vi "Multi Publisher.vi"() -> ()   [LabVIEW 2021]
uses:
  New Connection Request.ctl
  CIFChannels/CIFChannels.lvclass
  CIF_NIChn/FIFO_DAQ/CIF_NIChn_Fifo_DAQ.lvclass
  D:/dev/Packages/Channel_Manager/src/CIFChannels/CIFChannels.lvclass
  D:/dev/Packages/Channel_Manager/src/CIF_NIChn/NIChn/CIF_NIChn.lvclass
  CIFChannels/Typedef/Direction.ctl
  ChannelCommon/typedef/FIFO Config.ctl
  CIFChannels/CIFChannels.lvclass/CIFChannels.ctl
  ChannelCommon/typedef/Datatype Waveform.ctl
  ChannelCommon/typedef/TimeStamps.ctl
  CIF_NIChn/FIFO_DAQ/CIF_NIChn_Fifo_DAQ.lvclass/CIF_NIChn_Fifo_DAQ.ctl
  CIF_NIChn/NIChn/CIF_NIChn.lvclass/CIF_NIChn.ctl
  CIFChannels/Accessors/Write FIFO Retry on Timeout.vi
  CIFChannels/Accessors/Read Name.vi
  <vilib>/CIF Foundation/CIF Utilities/DataTypes/Flatten U64.vi
  CIF_NIChn/FIFO_DAQ/SubVIs/Core Write DAQ FIFO.vi
  ChannelCommon/Utilities/Reset Waveform DVRs.vi
  CIF_NIChn/FIFO_DAQ/SubVIs/Core Write DAQ DVR FIFO.vi
  ChannelCommon/Utilities/Get Waveform DVRs.vi
  CIFChannels/Accessors/Read FIFO Retry on Timeout.vi
  <vilib>/CIF Foundation/CIF Channels/CIFChannels/Top Level/Write U8 Array.vi
  CIF_NIChn/NIChn/Accessors/Read CIF Channel.vi
  CIF_NIChn/NIChn/Accessors/Write CIF Channel.vi
  CIF_NIChn/FIFO_DAQ/SubVIs/Flatten.vi
  CIFChannels/Accessors/Read FIFO Header.vi
  <vilib>/CIF Foundation/CIF Channels/CIFChannels/SubVIs/Get dll Path.vi
  <vilib>/CIF Foundation/CIF Channels/CIFChannels/SubVIs/Get Requested Size.vi
  ChannelCommon/CIFFIFO/Flatten/DVR Flatten.vi
  CIFChannels/Utilities/Create Flattened FIFO Header.vi
  ChannelCommon/Utilities/Flatten Header.vi
  CIFChannels/Utilities/Update FIFO Header.vi
  <vilib>/CIF Foundation/CIF Utilities/DataTypes/Flatten I64.vi
  <vilib>/CIF Foundation/CIF Utilities/Time/System Time/Get System Time.vi
  <vilib>/CIF Foundation/CIF Utilities/Time/System Time/LabVIEW Time to TAI Time.vi
  ChannelCommon/ChannelCommon.lvlib
panel:
  in  "Remove Pub":string
  in  "Remove":bool
  in  "stop":bool
  in  "Add":bool
  in  "New Sub":T1
  out "New Pub":string
  out "error out":errorcluster
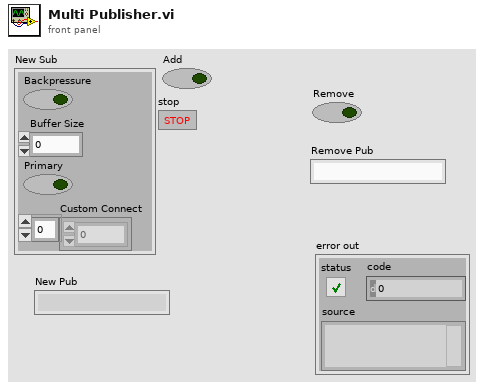
[diagram p1: front panel]
types:
  T1 = typedef "New Connection Request.ctl" = cluster{"Backpressure":bool, "Buffer Size":u64, "Primary":bool, "Custom Connect":u8[]}
  T2 = typedef "ChannelCommon.lvlib/TimeStamps.ctl" = cluster{"ClockID":u8, "T0":i64, "T_Out":i64}
  T3 = typedef "ChannelCommon.lvlib/Datatype Waveform.ctl" = cluster{"measurement":dbl[], "dT":dbl, "Timestamp":i64, "Read Lock":bool}
  T4 = typedef "ChannelCommon.lvlib/FIFO Config.ctl" = cluster{"Max Bytes/Msg":u64, "Max Msg/FIFO":u64, "Flags":u64}
  T5 = typedef "CIFChannels.lvclass/Direction.ctl" = enum16{"Publisher", "Subscriber"}
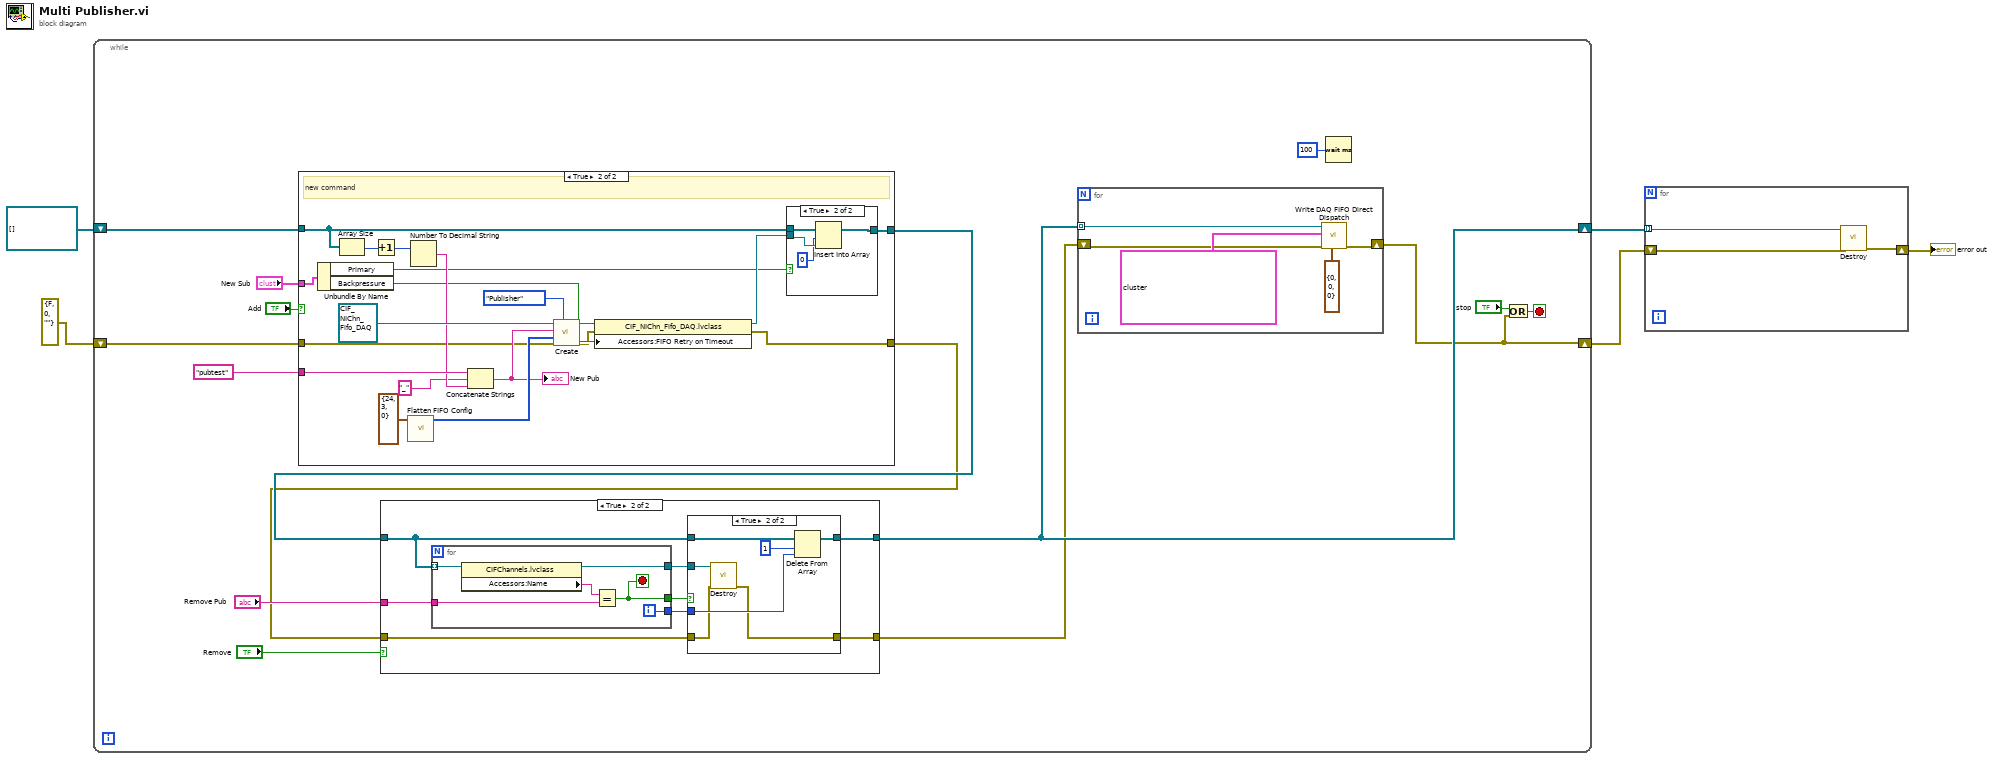
[diagram p0: block diagram]
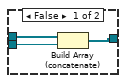
[diagram p5: hidden frame]
diagram:
  n1 = while {
    shift-right: [w12] -> w5
    shift-left: refnum<class "CIFChannels.lvclass">[] [] -> [w20]
    shift-right: [w7] -> w3
    shift-left: errorcluster {"status"=FALSE, "code"=0, "source"=""} ("error in (no error)") -> [w11]
    stop <- w6 stop-if-true
    n2 = case shown="True" "Add" {
      tunnel: "New Sub" -> [_ w72]
      tunnel: w20 -> [w52 w60]
      tunnel: "pubtest" -> [_ w67]
      tunnel: [w52 w58] -> w13
      tunnel: w11 -> [w51 w61]
      tunnel: [w51 w54] -> w10
      frame False {
        # "timedout"
      }
      frame True {
        # "new command"
        n3 = Unbundle By Name(w72) -> ("Primary"=w53:bool, "Backpressure"=w57:bool)
        n4 = Array Size(array=w60) -> (size(s)=w69:i32)
        n5 = Increment(x=w69) -> (x+1=w68:i32)
        n6 = call "Flatten FIFO Config.vi"("FIFO Config in"=T4 {"Max Bytes/Msg"=24, "Max Msg/FIFO"=3, "Flags"=0}) -> ("Flattened FIFO Config"=w63:u8[])  [unwired: 10 in]
        n7 = Number To Decimal String(number=w68) -> (decimal integer string=w66:string)  [unwired: 1 in]
        n8 = Concatenate Strings(w67, "_", w66) -> (w62:string)
        "New Pub" <- w62
        n9 = call-dynamic "Create.vi"("Direction"=Direction."Publisher", "error in (no error)"=w61, "Custom Config Data"=w63, "Name"=w62, "CIFTag in"=refnum<class "CIF_NIChn_Fifo_DAQ.lvclass"> refnum ("CIF_NIChn_Fifo_Power.lvclass")) -> ("error out"=w55:errorcluster, "CIFTag out"=w59:refnum<class "CIF_NIChn_Fifo_DAQ.lvclass">)  [unwired: 5 in]
        n10 = property class="CIF_NIChn_Fifo_DAQ.lvclass"(reference=w59, error in=w55, "Accessors:FIFO Retry on Timeout"=w57) -> (reference out=w56:refnum<class "CIF_NIChn_Fifo_DAQ.lvclass">, error out=w54:errorcluster)
        n11 = case shown="True" w53 {
          tunnel: w60 -> [w75 w79]
          tunnel: [w74 w76] -> w58
          tunnel: w56 -> [w73 w78]
          frame False {
            n12 = Build Array (concatenate)(w75, w73) -> (w74:refnum<class "CIFChannels.lvclass">[])
          }
          frame True {
            n13 = Insert Into Array(array=w79, index=0, new element=w78) -> (w76:refnum<class "CIFChannels.lvclass">[])
          }
        }
      }
    }
    n14 = case shown="True" "Remove" {
      tunnel: "Remove Pub" -> [_ w30]
      tunnel: w13 -> [w22 w29]
      tunnel: [w22 w23] -> w12
      tunnel: w10 -> [w21 w25]
      tunnel: [w21 w24] -> w9
      frame False {
      }
      frame True {
        n15 = for {
          tunnel: w29 -> [w45] mode=indexing
          tunnel: w30 -> [w43]
          tunnel: [w42] -> w28
          tunnel: [w41] -> w27
          tunnel: [w40] -> w26
          i -> [w40]
          stop <- w41 stop-if-true
          n16 = property class="CIFChannels.lvclass"(reference=w45) -> (reference out=w42:refnum<class "CIFChannels.lvclass">, "Accessors:Name"=w44:string)  [unwired: 1 in, 1 out]
          n17 = Equal?(x=w44, y=w43) -> (x = y?=w41:bool)
        }
        n18 = case shown="True" w27 {
          tunnel: w29 -> [w31 w39]
          tunnel: w28 -> [_ w38]
          tunnel: w26 -> [_ w37]
          tunnel: w25 -> [w32 w35]
          tunnel: [w32 w34] -> w24
          tunnel: [w31 w33] -> w23
          frame False {
          }
          frame True {
            n19 = call-dynamic "Destroy.vi"("error in (no error)"=w35, "CIFChannels in"=w38) -> ("error out"=w34:errorcluster)  [unwired: 8 in, 1 out]
            n20 = Delete From Array(array=w39, length=1, index=w37) -> (array with subset deleted=w33:refnum<class "CIFChannels.lvclass">[])  [unwired: 1 out]
          }
        }
      }
    }
    n21 = for {
      tunnel: w12 -> [w46] mode=indexing
      shift-right: [w48] -> w7
      shift-left: w9 -> [w49]
      n22 = call "Write DAQ FIFO Direct Dispatch.vi"("FIFO Timestamps"=T2 {"ClockID"=0, "T0"=0, "T_Out"=0}, "error in (no error)"=w49, "DAQ In"=T3[] [{"measurement"=array[986 elements], "dT"=43.0, "Timestamp"=2, "Read Lock"=FALSE}, {"measurement"=array[1001 elements], "dT"=34.0, "Timestamp"=1, "Read Lock"=FALSE}], "CIFTag in"=w46) -> ("error out"=w48:errorcluster)  [unwired: 4 in, 3 out]
    }
    n23 = Wait (ms)(milliseconds to wait=u32 100) -> ()  [unwired: 1 out]
    n24 = Or(x="stop", y=w7) -> (x .or. y?=w6:bool)
  }
  n25 = for {
    tunnel: w5 -> [w80] mode=indexing
    shift-right: [w81] -> w2
    shift-left: w3 -> [w82]
    n26 = call-dynamic "Destroy.vi"("error in (no error)"=w82, "CIFChannels in"=w80) -> ("error out"=w81:errorcluster)  [unwired: 8 in, 1 out]
  }
  "error out" <- w2
